vi "Write.vi"(9 "Data":u8 format="%02x", 10 "Address":u16 format="%04x", 11 "EEPROM in":refnum<class "EEPROM.lvclass">) -> (3 "EEPROM out":refnum<class "EEPROM.lvclass">)   [LabVIEW 2021, in "EEPROM.lvclass"]
uses:
  EEPROM.lvclass
  EEPROM.lvclass/EEPROM.ctl
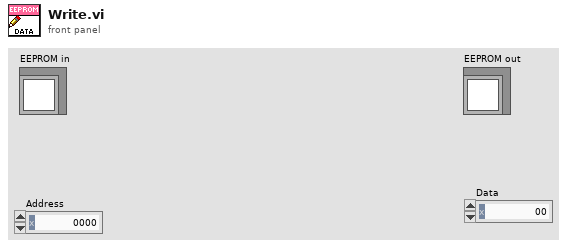
[diagram p1: front panel]
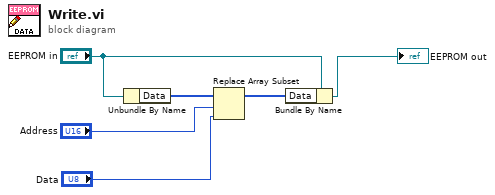
[diagram p0: block diagram]
diagram:
  n1 = Unbundle By Name("EEPROM in") -> ("Data"=w6:u8[])
  n2 = Replace Array Subset(array=w6, new element="Data", index="Address") -> (w3:u8[])
  n3 = Bundle By Name(cluster="EEPROM in", "Data"=w3) -> (→"EEPROM out":refnum<class "EEPROM.lvclass">)
